vi "PostScanAction.vi"(0 "Device en entrée":refnum<class "MultiHarp150.lvclass"> caption="DNL_LabVIEW Object in", 5 "AcqComp":bool, 7 "ScanDev":bool caption="AcqComp", 11 "error in (no error)":errorcluster caption="entrée d'erreur (pas d'erreur)") -> (4 "Device en sortie":refnum<class "MultiHarp150.lvclass"> caption="DNL_LabVIEW Object out", 6 "PostScanString":string, 15 "error out":errorcluster caption="sortie d'erreur")   [LabVIEW 2019, in "MultiHarp150.lvclass"]
uses:
  MultiHarp150.lvclass
  MultiHarp150.lvclass/MultiHarp150.ctl
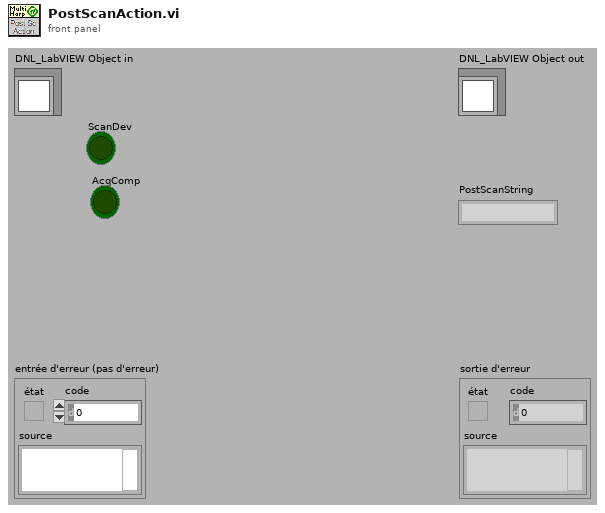
[diagram p1: front panel]
types:
  T1 = cluster{"TagIdent":string, "TagIndex":i32, "TagType":i32, "TagValue":i64, "TagAuxData":string}[]
  T2 = typedef "MultiHarp150.lvclass/MultiHarp150_Func.ctl" = enum16{"ReadHistogram (Ph)", "ReadT2 (Ph)", "ReadT3 (Ph)", "ReadCount (Ph)"}
  T3 = cluster{"TagIdent":string, "TagIndex":i32, "TagType":i32, "TagValue":i64, "TagAuxData":string}
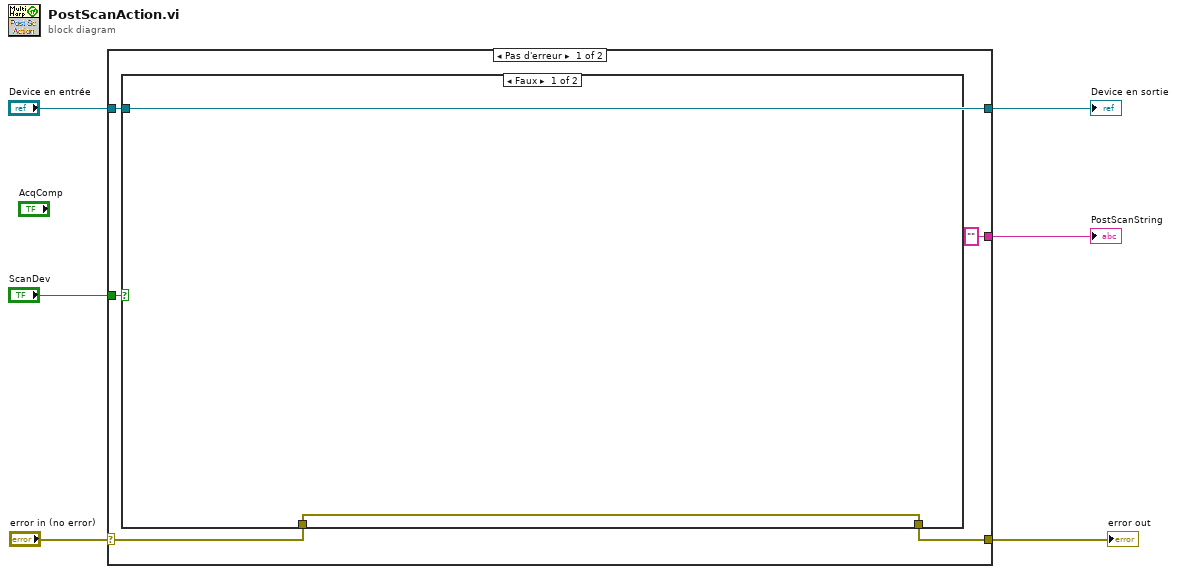
[diagram p0: block diagram]
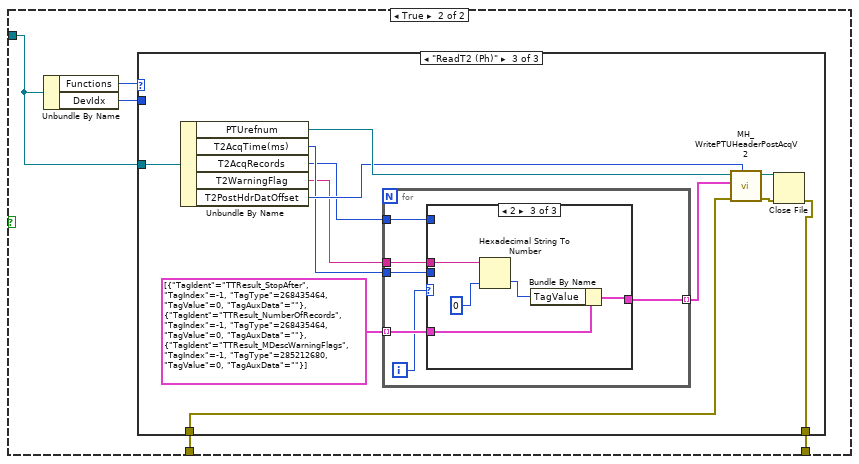
[diagram p2: hidden frame]
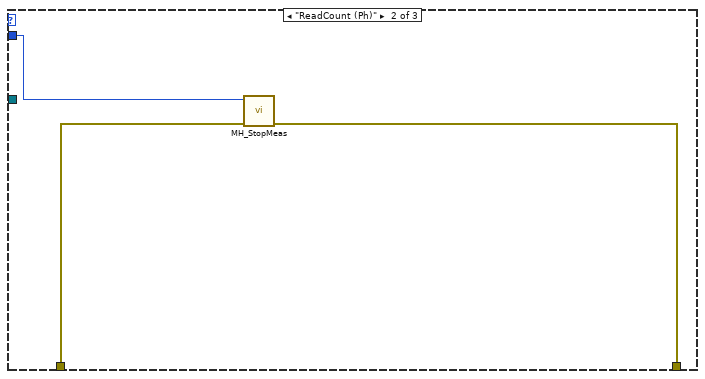
[diagram p4: hidden frame]
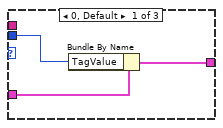
[diagram p5: hidden frame]
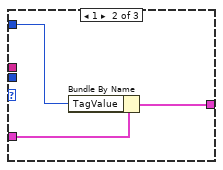
[diagram p6: hidden frame]
diagram:
  n1 = case shown="Pas d'erreur" "error in (no error)" {
    selector: "error in (no error)" -> [w10 w52]
    tunnel: [w9 w52] -> w2
    tunnel: [w8 w51] -> w5
    tunnel: "Device en entrée" -> [w8 w51]
    tunnel: ["" _] -> w4
    tunnel: "ScanDev" -> [w7 _]
    frame No Error {
      n2 = case shown="Faux" w7 {
        tunnel: w10 -> [w12 w17]
        tunnel: [w12 w16] -> w9
        tunnel: w8 -> [_ w15]
        frame False {
        }
        frame True {
          n3 = Unbundle By Name(w15) -> ("Functions"=w14:T2, "DevIdx"=w13:i32)
          n4 = case shown="\"ReadT2 (Ph)\"" w14 {
            tunnel: w17 -> [w18 w20 w27]
            tunnel: [w18 w19 w22] -> w16
            tunnel: w15 -> [_ _ w25]
            tunnel: w13 -> [_ w21 _]
            frame "ReadHistogram (Ph)", Default {
            }
            frame "ReadCount (Ph)" {
              n5 = call <userlib>:"MH_StopMeas.vi"("error in (no error)"=w20, "devidx"=w21) -> ("error out"=w19:errorcluster)  [unwired: 8 in, 1 out]
            }
            frame "ReadT2 (Ph)" {
              n6 = Unbundle By Name(w25) -> ("PTUrefnum"=w33:refnum<file>, "T2AcqTime(ms)"=w30:u32, "T2AcqRecords"=w26:i64, "T2WarningFlag"=w29:string, "T2PostHdrDatOffset"=w32:i64)
              n7 = for {
                tunnel: T1 [{"TagIdent"="TTResult_StopAfter", "TagIndex"=-1, "TagType"=268435464, "TagValue"=0, "TagAuxData"=""}, {"TagIdent"="TTResult_NumberOfRecords", "TagIndex"=-1, "TagType"=268435464, "TagValue"=0, "TagAuxData"=""}, {"TagIdent"="TTResult_MDescWarningFlags", "TagIndex"=-1, "TagType"=285212680, "TagValue"=0, "TagAuxData"=""}] ("sous-tableau") -> [w39] mode=indexing
                tunnel: w30 -> [w38]
                tunnel: w29 -> [w37]
                tunnel: [w36] -> w28 mode=indexing
                tunnel: w26 -> [w34]
                i -> [w35]
                n8 = case shown="2" w35 {
                  tunnel: w39 -> [w42 w45 w46]
                  tunnel: w38 -> [w41 _ _]
                  tunnel: w37 -> [_ _ w49]
                  tunnel: [w40 w44 w48] -> w36
                  tunnel: w34 -> [_ w43 _]
                  frame 0, Default {
                    n9 = Bundle By Name(cluster=w42, "TagValue"=w41) -> (w40:T3)
                  }
                  frame 1 {
                    n10 = Bundle By Name(cluster=w45, "TagValue"=w43) -> (w44:T3)
                  }
                  frame 2 {
                    n11 = Hexadecimal String To Number(string=w49, default (0uL)=i64 0 ("TagValue")) -> (number=w47:i64)  [unwired: 1 in, 1 out]
                    n12 = Bundle By Name(cluster=w46, "TagValue"=w47) -> (w48:T3)
                  }
                }
              }
              n13 = call <userlib>:"MH_WritePTUHeaderPostAcqV2.vi"("FileOffset(bytes)"=w32, "entrée d'erreur"=w27, "TagArray"=w28, "refnum In"=w33) -> ("sortie d'erreur"=w24:errorcluster, "refnum Out"=w23:refnum<file>)  [unwired: 6 in]
              n14 = Close File(refnum=w23, error in=w24) -> (error out=w22:errorcluster)  [unwired: 1 out]
            }
          }
        }
      }
    }
    frame Error {
    }
  }
  "error out" <- w2
  "Device en sortie" <- w5
  "PostScanString" <- w4
